vi "RxCalOn.vi"(8 "error in (no error)":errorcluster, 11 "RxCalConfig":T1) -> (0 "error out":errorcluster)   [LabVIEW 2015]
uses:
  RXCalDLL.dll
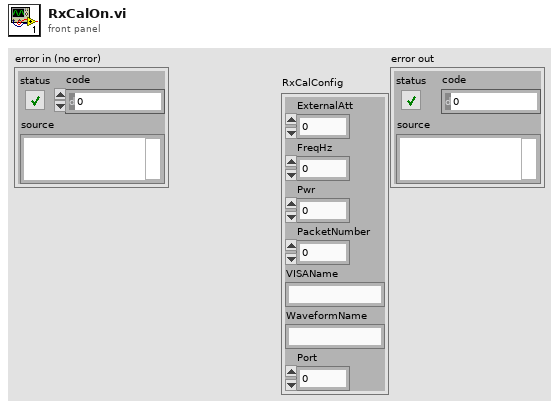
[diagram p1: front panel]
types:
  T1 = cluster{"ExternalAtt":dbl, "FreqHz":dbl, "Pwr":dbl, "PacketNumber":i32, "VISAName":string, "WaveformName":string, "Port":u32}
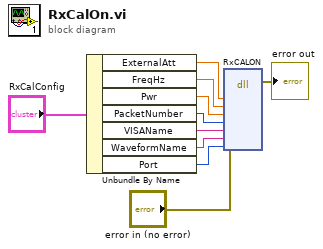
[diagram p0: block diagram]
diagram:
  n1 = Unbundle By Name("RxCalConfig") -> ("ExternalAtt"=w9:dbl, "FreqHz"=w8:dbl, "Pwr"=w7:dbl, "PacketNumber"=w6:i32, "VISAName"=w5:string, "WaveformName"=w4:string, "Port"=w3:u32)
  n2 = dll-call lib="D:/4-Up-WLAN-Test-System/WTSInstrumentControl/rx cal/RXCalDLL.dll" fn="RxCALON"(error in="error in (no error)", "ExternalAtt"=w9, "FreqHz"=w8, "Pwr"=w7, "PacketNumber"=w6, "VISAName"=w5, "WaveformName"=w4, "Port"=w3) -> (error out=→"error out":errorcluster)  [unwired: 10 in, 1 out]
